vi "Create_Directory.vi"(0 "Test":string, 3 "PMTs":string[](array[string])) -> (7 "Paths":path[](array[path]), 10 "File exists":bool)   [LabVIEW 2018]
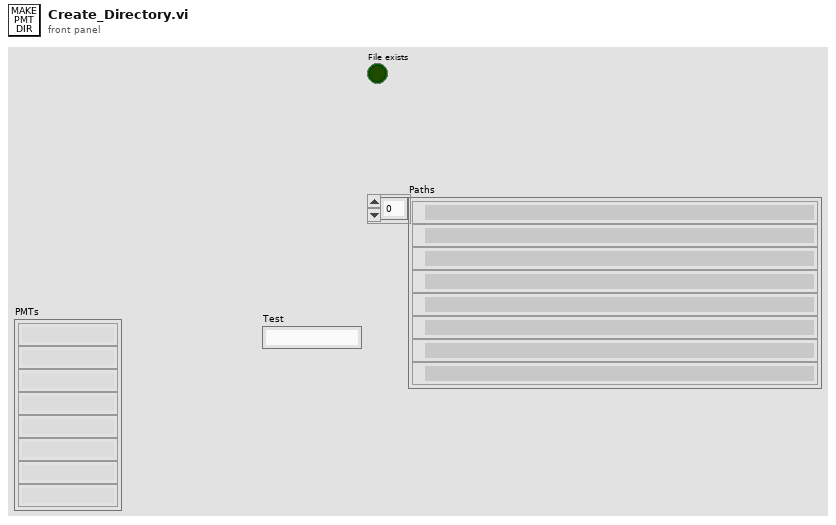
[diagram p1: front panel]
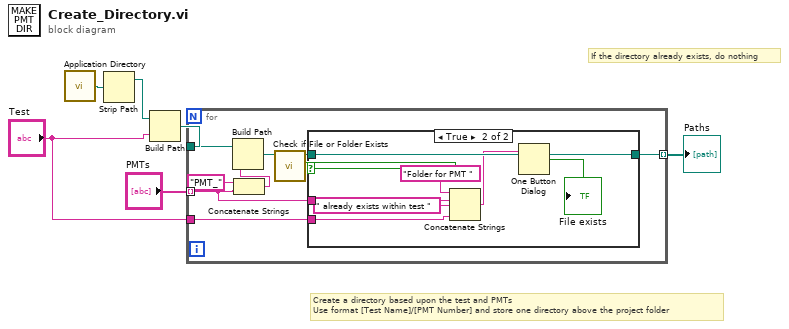
[diagram p0: block diagram]
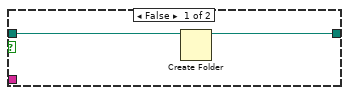
[diagram p2: hidden frame]
diagram:
  # "If the directory already exists, do nothing"
  # "Create a directory based upon the test and PMTs\nUse format [Test Name]/[PMT Number] and store one directory above the project folder"
  n1 = call <vilib>:"Application Directory.vi"() -> ("Application Directory"=w5:path)
  n2 = Strip Path(path=w5) -> (stripped path=w6:path)  [unwired: 1 out]
  n3 = Build Path(base path=w6, name or relative path="Test") -> (appended path=w3:path)
  n4 = for {
    tunnel: "PMTs" -> [w9] mode=indexing
    tunnel: [w13] -> w4 mode=indexing
    tunnel: w3 -> [w12]
    tunnel: "Test" -> [w10]
    n5 = Concatenate Strings("PMT_" ("string"), w9) -> (w8:string)
    n6 = Build Path(base path=w12, name or relative path=w8) -> (appended path=w11:path)
    n7 = call <vilib>:"Check if File or Folder Exists.vi"("path"=w11) -> ("file or folder exists?"=w15:bool, "dup path"=w14:path)  [unwired: 8 in, 1 out]
    n8 = case shown="True" w15 {
      tunnel: w14 -> [w17 w24]
      tunnel: [w16 w24] -> w13
      tunnel: w9 -> [_ w21]
      tunnel: w10 -> [_ w19]
      frame False {
        n9 = Create Folder(path (use dialog)=w17) -> (created path=w16:path)  [unwired: 2 in, 2 out]
      }
      frame True {
        n10 = Concatenate Strings("Folder for PMT " ("message"), w21, " already exists within test " ("string"), w19) -> (w23:string)
        n11 = One Button Dialog(message=w23) -> (true=→"File exists":bool)  [unwired: 1 in]
      }
    }
  }
  "Paths" <- w4
